vi "GUI_HTU_Control_Center.vi"() -> ()   [LabVIEW 2020]
uses:
  Shared/GUI_Template/GUI_master/tcp_new_data_event.ctl
  Shared/GUI_Template/GUI_master/tcp new data cluster.ctl
  GUI_TestStand/Fire button.ctl
panel:
  in  "Position.Ch1::36":dbl caption="TC Out Stage" min=0.0 max=12.0
  in  "Position.Ch2::36":dbl caption="TC In Stage" min=0.0 max=12.0
  in  "GUIdevice 36":string="U_EMQTripletBipolar"
  in  "DO.Ch21::22":enum16{"off", "on"}(ring) caption="UV spec\nmirror"
  in  "gaia shutter B":bool caption="Gaia internal\nshutter B"
  in  "gaia shutter A":bool caption="Gaia internal \nshutter A"
  in  "DO.Ch20::22":enum16{"off", "on"}(ring) caption="UV spec\nprotector"
  in  "Current_Limit.Ch4::35":dbl caption="BCave Trim\nCurrent" min=0.0 max=12.0
  in  "GUIdevice 35":string="U_EMQTripletBipolar"
  in  "Current::34":dbl caption="ACave \nCurrent" min=-40.0 max=40.0
  in  "Current_Limit.Ch1::33":dbl caption="BCave \nCurrent" min=0.0 max=120.0
  in  "GUIdevice 34":string="U_ACaveMagSpecPS"
  in  "GUIdevice 33":string="U_BCaveMagSpecPS"
  out "Rawfield::32":dbl caption="ACave Hall \nprobe" min=0.0 max=0.0
  in  "GUIdevice 32":string="U_ACaveHallProbe"
  out "Rawfield::31":dbl caption="BCave Hall \nprobe" min=0.0 max=0.0
  in  "GUIdevice 31":string="U_BCaveHallProbe"
  in  "Amplitude.Ch AB::30":dbl caption="Amplitude Jet trigger" min=0.5 max=5.0 format="%.1f"
  out "Amplitude.Ch AB::30":dbl caption="Amplitude\n Jet trigger" min=0.5 max=5.0 format="%.1f"
  in  "MRC trigger":bool caption="MRC \nTrigger"
  in  "GUIdevice 30":string="U_MRC_TimingBox"
  out "Internal Shutter B":string
  out "Internal Shutter A":string
  out "PockelCellB::29":dbl caption="pockelcellB" min=0.0 max=0.0 format="%.3f"
  out "pockelcella::29":dbl caption="pockelcellA" min=0.0 max=0.0 format="%.3f"
  in  "internalshutterb::29":dbl caption="Internal Shutter B" min=0.0 max=0.0 format="%.3f"
  in  "internalshuttera::29":dbl caption="Internal Shutter A" min=0.0 max=0.0 format="%.3f"
  in  "GUIdevice 29":string="U_GaiaSVEReader"
  in  "delay.Channel_C::18":dbl caption="Gaia lamp timing" min=-1.0 max=1.0
  in  "GUIdevice 18":string="U_1HzShiftedBox"
  in  "Position.Ch3::26":dbl caption="Ghost\nfilter" min=0.0 max=100.0
  in  "Position.Ch2::26":dbl caption="Ghost\nfocus" min=0.0 max=100.0
  in  "GUIdevice 15":string="U_MI_CoarseFilters"
  in  "GUIdevice 14":string="U_HASO_Filters"
  in  "GUIdevice 9":string="U_ProbeFilters"
  in  "DO.Ch11::22":enum16{"off", "on"}(ring) caption="TC phos"
  in  "GUIdevice 28":string="U_MI_FineFilters"
  in  "pos.Channel0::28":enum16{"1", "2", "3", "4", "5", "6"}(ring) caption="Fine Filters"
  in  "DO.Ch9::22":enum16{"off", "on"}(ring) caption="Aline2"
  in  "SoftwareVars.Ch1::22":enum16{"off", "on"}(ring) caption="Autopurge"
  in  "DO.Ch8::22":enum16{"off", "on"}(ring) caption="Aline 3"
  in  "DO.Ch7::22":enum16{"off", "on"}(ring) caption="DC Phos"
  in  "auto purge":bool=TRUE
  in  "purge":bool caption="Purge"
  in  "DO.Ch6::22":enum16{"off", "on"}(ring) caption="purge"
  in  "Offset::20":dbl caption="Probe cam\noffset" min=-40.0 max=40.0 format="%#_3g"
  out "AI_mean.Channel 1::27":dbl caption="Energy (nJ)" min=0.0 max=0.0 format="%.3f"
  out "AI_mean.Channel 0::27":dbl caption="Energy (nJ)" min=0.0 max=0.0 format="%.3f"
  in  "GUIdevice 27":string="U_VacuumGauge"
  out "ACavePressure":dbl format="%#_3g"
  out "BCavePressure":dbl format="%#_3g"
  in  "DO.Ch19::22":enum16{"off", "on"}(ring) caption="Visa9"
  in  "Position.Ch1::26":dbl caption="Phasics\nfocus" min=0.0 max=99.0
  in  "GUIdevice 26":string="U_Zaber"
  in  "DigitalOutput.Channel 7::25":enum16{"off", "on"}(ring) caption="Visa1"
  in  "DigitalOutput.Channel 6::25":enum16{"off", "on"}(ring) caption="Visa2"
  in  "DigitalOutput.Channel 5::25":enum16{"off", "on"}(ring) caption="Visa3"
  in  "DigitalOutput.Channel 4::25":enum16{"off", "on"}(ring) caption="Visa4"
  in  "DigitalOutput.Channel 3::25":enum16{"off", "on"}(ring) caption="Visa5"
  in  "DigitalOutput.Channel 2::25":enum16{"off", "on"}(ring) caption="Visa6"
  in  "DigitalOutput.Channel 1::25":enum16{"off", "on"}(ring) caption="Visa7"
  in  "DigitalOutput.Channel 0::25":enum16{"off", "on"}(ring) caption="Visa8"
  in  "GUIdevice 25":string="U_VisaPlungers"
  in  "DO.Ch18::22":enum16{"off", "on"}(ring) caption="Aline1"
  in  "GUIdevice 23":string="U_SSR_2"
  in  "DO.Ch5::22":enum16{"off", "on"}(ring) caption="Beam \nDump"
  in  "DO.Ch4::22":enum16{"off", "on"}(ring) caption="Phos1"
  in  "DO.Ch3::22":enum16{"off", "on"}(ring) caption="MI Wedge"
  in  "DO.Ch2::22":enum16{"off", "on"}(ring) caption="Slit"
  in  "DO.Ch1::22":enum16{"off", "on"}(ring) caption="OAPin2"
  in  "GUIdevice 22":string="U_PLC"
  in  "GUIdevice 21":string="U_BCavePicoServer"
  in  "Position::20":dbl caption="Probe cam\nStage" min=-25.0 max=25.0 format="%#_3g"
  in  "GUIdevice 20":string="U_ProbeCamStage"
  in  "Position.Axis 6::16":dbl caption="DM Surf. Y" min=1.9 max=3.0
  in  "Position.Axis 5::16":dbl caption="DM Surf. X" min=1.5 max=3.1
  in  "pos.Channel0::14":enum16{"1", "2", "3", "4", "5", "6"}(ring) caption="HASO"
  in  "pos.Channel0::19":enum16{"1", "2", "3", "4", "5", "6"}(ring) caption="Grating \nCam"
  in  "GUIdevice 19":string="U_FilterWheel_02"
  in  "Delay.Ch B::10":dbl caption="OPening time" min=0.0 max=0.1 format="%#_6p"
  in  "Amplitude.Ch AB::10":dbl caption="Amplitude Jet trigger" min=0.5 max=5.0 format="%.1f"
  in  "DO.Ch10::22":enum16{"off", "on"}(ring) caption="CTR"
  in  "GUIdevice 17":string="U_Hexapod"
  out "Position.Axis2::11":dbl caption="Angle 1" min=-180.0 max=180.0
  out "Position.Axis3::11":dbl caption="Angle 2" min=-180.0 max=180.0
  in  "Position.Axis 4::16":dbl caption="OAP1 In Y" min=2.0 max=5.0
  in  "Position.Axis 3::16":dbl caption="OAP1 In X" min=2.25 max=3.3
  in  "Position.Axis 2::16":dbl caption="BCave In Y" min=2.5 max=3.5
  in  "Position.Axis 1::16":dbl caption="BCave In X" min=2.0 max=4.0
  in  "GUIdevice 16":string="U_TRAServer03"
  in  "Position.Channel 9::1":T1(ring) caption="Amp 4 dump"
  in  "Position.Channel 10::1":T1(ring) caption="Gaia amp2 south energy"
  in  "Position.Axis 111::13":dbl caption="Blade Height" min=-999999.0 max=999999.0
  in  "GUIdevice 13":string="U_BCavePicoServer"
  in  "GUIdevice 12":string="U_TRAServer03"
  in  "Position.Channel 7::1":T1(ring) caption="Gaia Beamblock 2-North"
  in  "Position.Channel 8::1":T1(ring) caption="Gaia Beamblock 2-South"
  out "Delay.Ch B::10":dbl caption="Opening \ntime (s)" min=0.0 max=0.1 format="%#_6p"
  in  "Set opening time (s)":dbl
  in  "Jet enable":bool caption="Jet Enable"
  in  "Position.Axis 3::6":dbl caption="Probe \ndelay" min=0.0 max=25.0
  in  "Position.Axis 2::6":dbl caption="Jet Blade" min=-23.5 max=0.0
  in  "Position.Axis1::11":dbl caption="Separation" min=-60000.0 max=60000.0
  in  "GUIdevice 11":string="U_CompAerotech"
  in  "pos.Channel0::9":enum16{"1", "2", "3", "4", "5", "6"}(ring) caption="Probe"
  in  "pos.Channel0::5":enum16{"1", "2", "3", "4", "5", "6"}(ring) caption="Ghost\npulsed"
  in  "AnalogOutput.Channel 1::8":dbl caption="Pressure Control Voltage (V)" min=0.0 max=10.0
  in  "Position.Axis 3::7":dbl caption="Jet_Z" min=0.0 max=25.0
  in  "Position.Axis 2::7":dbl caption="Jet_Y" min=-25.0 max=0.0
  in  "Position.Axis 1::7":dbl caption="Jet_X" min=0.0 max=25.0
  in  "pos.Channel0::15":enum16{"1", "2", "3", "4", "5", "6"}(ring) caption="Coarse Filters"
  in  "Position.Channel 6::1":T1(ring) caption="Gaia Beamblock 3-North"
  in  "Position.Channel 5::1":T1(ring) caption="Gaia Beamblock 4-North"
  in  "Position.Channel 4::1":T1(ring) caption="Gaia Stop South"
  in  "Position.Channel 3::1":T1(ring) caption="Gaia Stop North"
  in  "Position.Channel 2::1":T1(ring) caption="Gaia Beamblock 3-South"
  in  "Position.Channel 1::1":T1(ring) caption="Gaia Beamblock 4-South"
  in  "Position.Axis 1::6":dbl caption="Position" min=-130.0 max=30.0
  in  "Position.Axis 6::4":dbl caption="Beamline In Y" min=1.5 max=2.9
  in  "Position.Axis 5::4":dbl caption="Beamline In X" min=2.5 max=4.0
  in  "Position.Axis 4::4":dbl caption="Beamline Out Y" min=2.6 max=3.2
  in  "Position.Axis 3::4":dbl caption="Beamline Out X" min=2.8 max=3.4
  in  "Position.Axis 2::4":dbl caption="OAP In 2 Y" min=2.5 max=3.3
  in  "Position.Axis 1::4":dbl caption="OAP In 2 X" min=3.1 max=3.6
  in  "Position.Axis 4::3":dbl caption="Comp In Y" min=5.5 max=5.9
  in  "Position.Axis 3::3":dbl caption="Comp In X" min=1.3 max=1.6
  in  "Position.Axis 2::3":dbl caption="Tube In Y" min=1.4 max=1.6
  in  "Position.Axis 1::3":dbl caption="Tube In X" min=1.2 max=1.4
  in  "GUIdevice 8":string="U_HP_Daq"
  in  "GUIdevice 6":string="U_ModeImagerESP"
  in  "GUIdevice 5":string="U_GhostFilters"
  in  "Fire Button":T2=TRUE
  out "error IO 2":errorcluster
  out "Amplitude.Ch AB::10":dbl caption="Amplitude\n Jet trigger" min=0.5 max=5.0 format="%.1f"
  out "fire::10":string
  out "tcp data event":T3
  in  "UDP error message":string
  in  "GUIdevice 7":string="U_ESP_JetXYZ"
  in  "GUIdevice 2":string="U_1Wire_Bcave"
  in  "GUIdevice 10":string="U_DG645_ShotControl"
  in  "GUIdevice 4":string="U_TRAServer02"
  in  "GUIdevice 1":string="U_1Wire_148"
  in  "GUIdevice 3":string="U_TRAServer01"
  in  "Step size":dbl min=-22.0 max=22.0 format="%.5f"
  in  "wangle::17":dbl caption="w" min=-7.5 max=7.5 step=0.01 format="%.5f"
  in  "vangle::17":dbl caption="v" min=-7.5 max=7.5 step=0.01 format="%.5f"
  in  "uangle::17":dbl caption="u" min=-7.5 max=7.5 step=0.01 format="%.5f"
  in  "ypos::17":dbl caption="y" min=-24.0 max=24.0 step=0.01 format="%.5f"
  in  "zpos::17":dbl caption="z" min=-10.0 max=10.0 step=0.01 format="%.5f"
  in  "xpos::17":dbl caption="x" min=-20.0 max=20.0 step=0.01 format="%.5f"
  in  "Jet trigger":bool caption="Jet Trigger"
  in  "Delay.Ch C::10":dbl caption="Jet timing (s)" min=-0.1 max=0.1 format="%#_6p"
  in  "stop":bool
  # "HTU CONTROL CENTER"
  # "Jet Stages"
  # "GAIA control"
  # "B-Cave Alignment"
  # "\"+x\" moves toward parking lot\n\"+y\" moves down\n\"+z\" moves upstream\n\"+\" moves jet blade out of jet\n\"+\" blade height moves away from jet"
  # "Mode Imager"
  # "Jet timing"
  # "Compressor"
  # "Hexapod"
  # "Misc area"
  # "148 TRA motors"
  # "\"+x\" is laser propagation direction\n\"+y\" is toward parking lot\n\"+z\" is up\nPMQ out at y=-22.0, in at ~17.5"
  # "\"in\" at position 0.0\n\"out\" at position 75.0"
  # "Vacuum"
  # "Valve Control"
  # "Extra Flippers"
  # "Mag Specs"
  # "Filters"
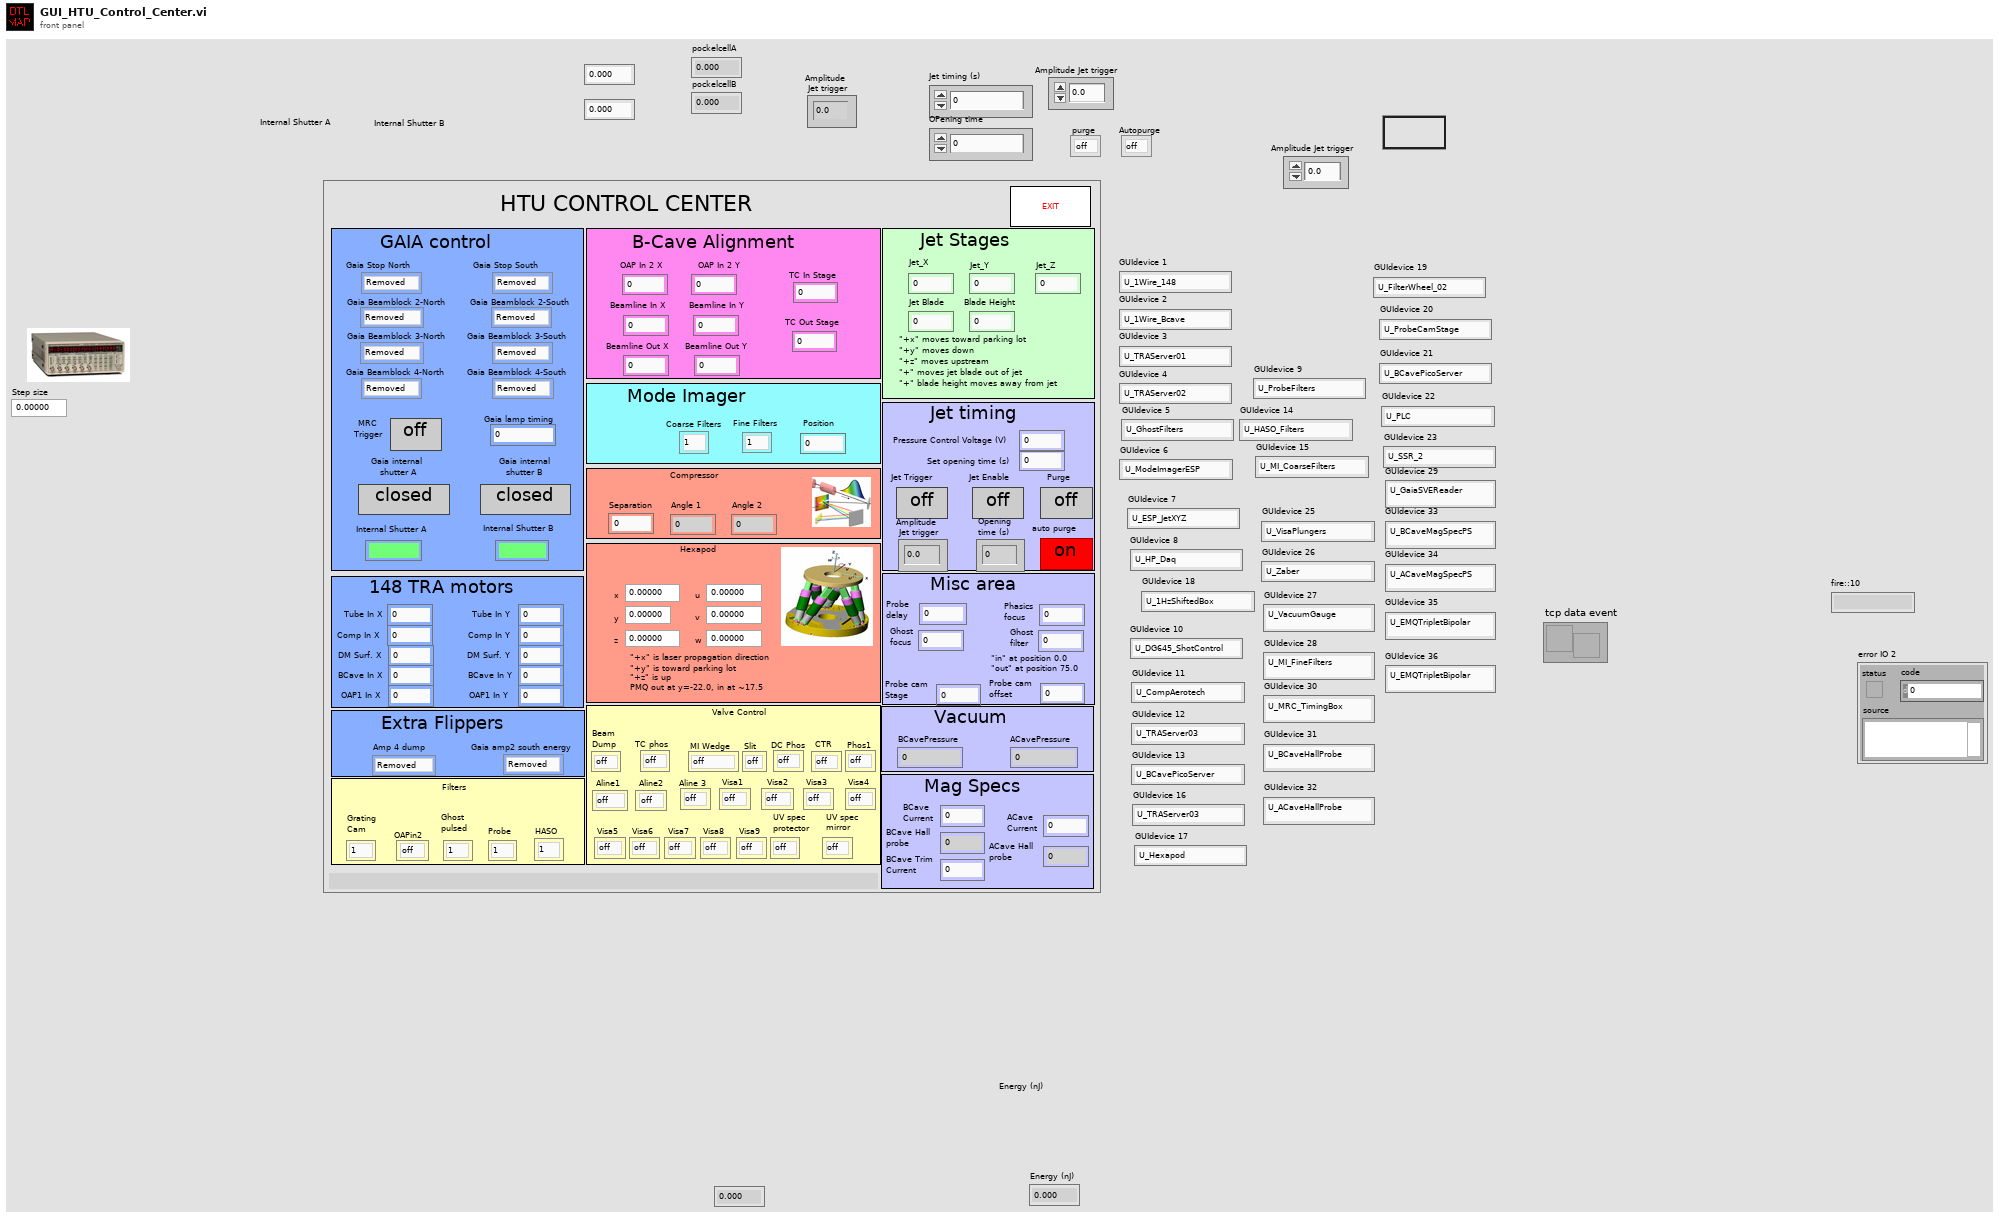
[diagram p1: front panel]
types:
  T1 = enum16{"Removed", "Inserted", "Unknown", "Moving"}
  T2 = typedef "Fire button.ctl" = bool
  T3 = typedef "tcp_new_data_event.ctl" = refnum<user-event>
  T4 = typedef "tcp new data cluster.ctl" = cluster{"EventEnum":enum16{"new data", "connection status update"}, "Device name":string}
  T5 = enum32{"invalid app kind", "Development System", "Run Time System", "Student Edition", "Embedded LabVIEW", "Evaluation", "Custom"}
  T6 = enum32{"Invalid", "Standard", "Closed", "Hidden", "Minimized", "Maximized"}
  T7 = cluster{"Core":cluster{"Current VI Reference":refnum<vi>, "Close Panel on Exit?":bool}, "BCavePressure":dbl, "ACavePressure":dbl, "Jet trigger":bool, "Jet probe stage tck":u32, "Tik2":u32, "Fire Continues Allowed":bool, "Jet enable":bool, "Wedge enable":bool, "Phosphor enable":bool, "jet status tck":i32, "purge":bool, "auto purge":bool, "MRC trigger":bool, "gaia shutter A":bool, "gaia shutter B":bool}
  T8 = cluster{"Current VI Reference":refnum<vi>, "Close Panel on Exit?":bool}
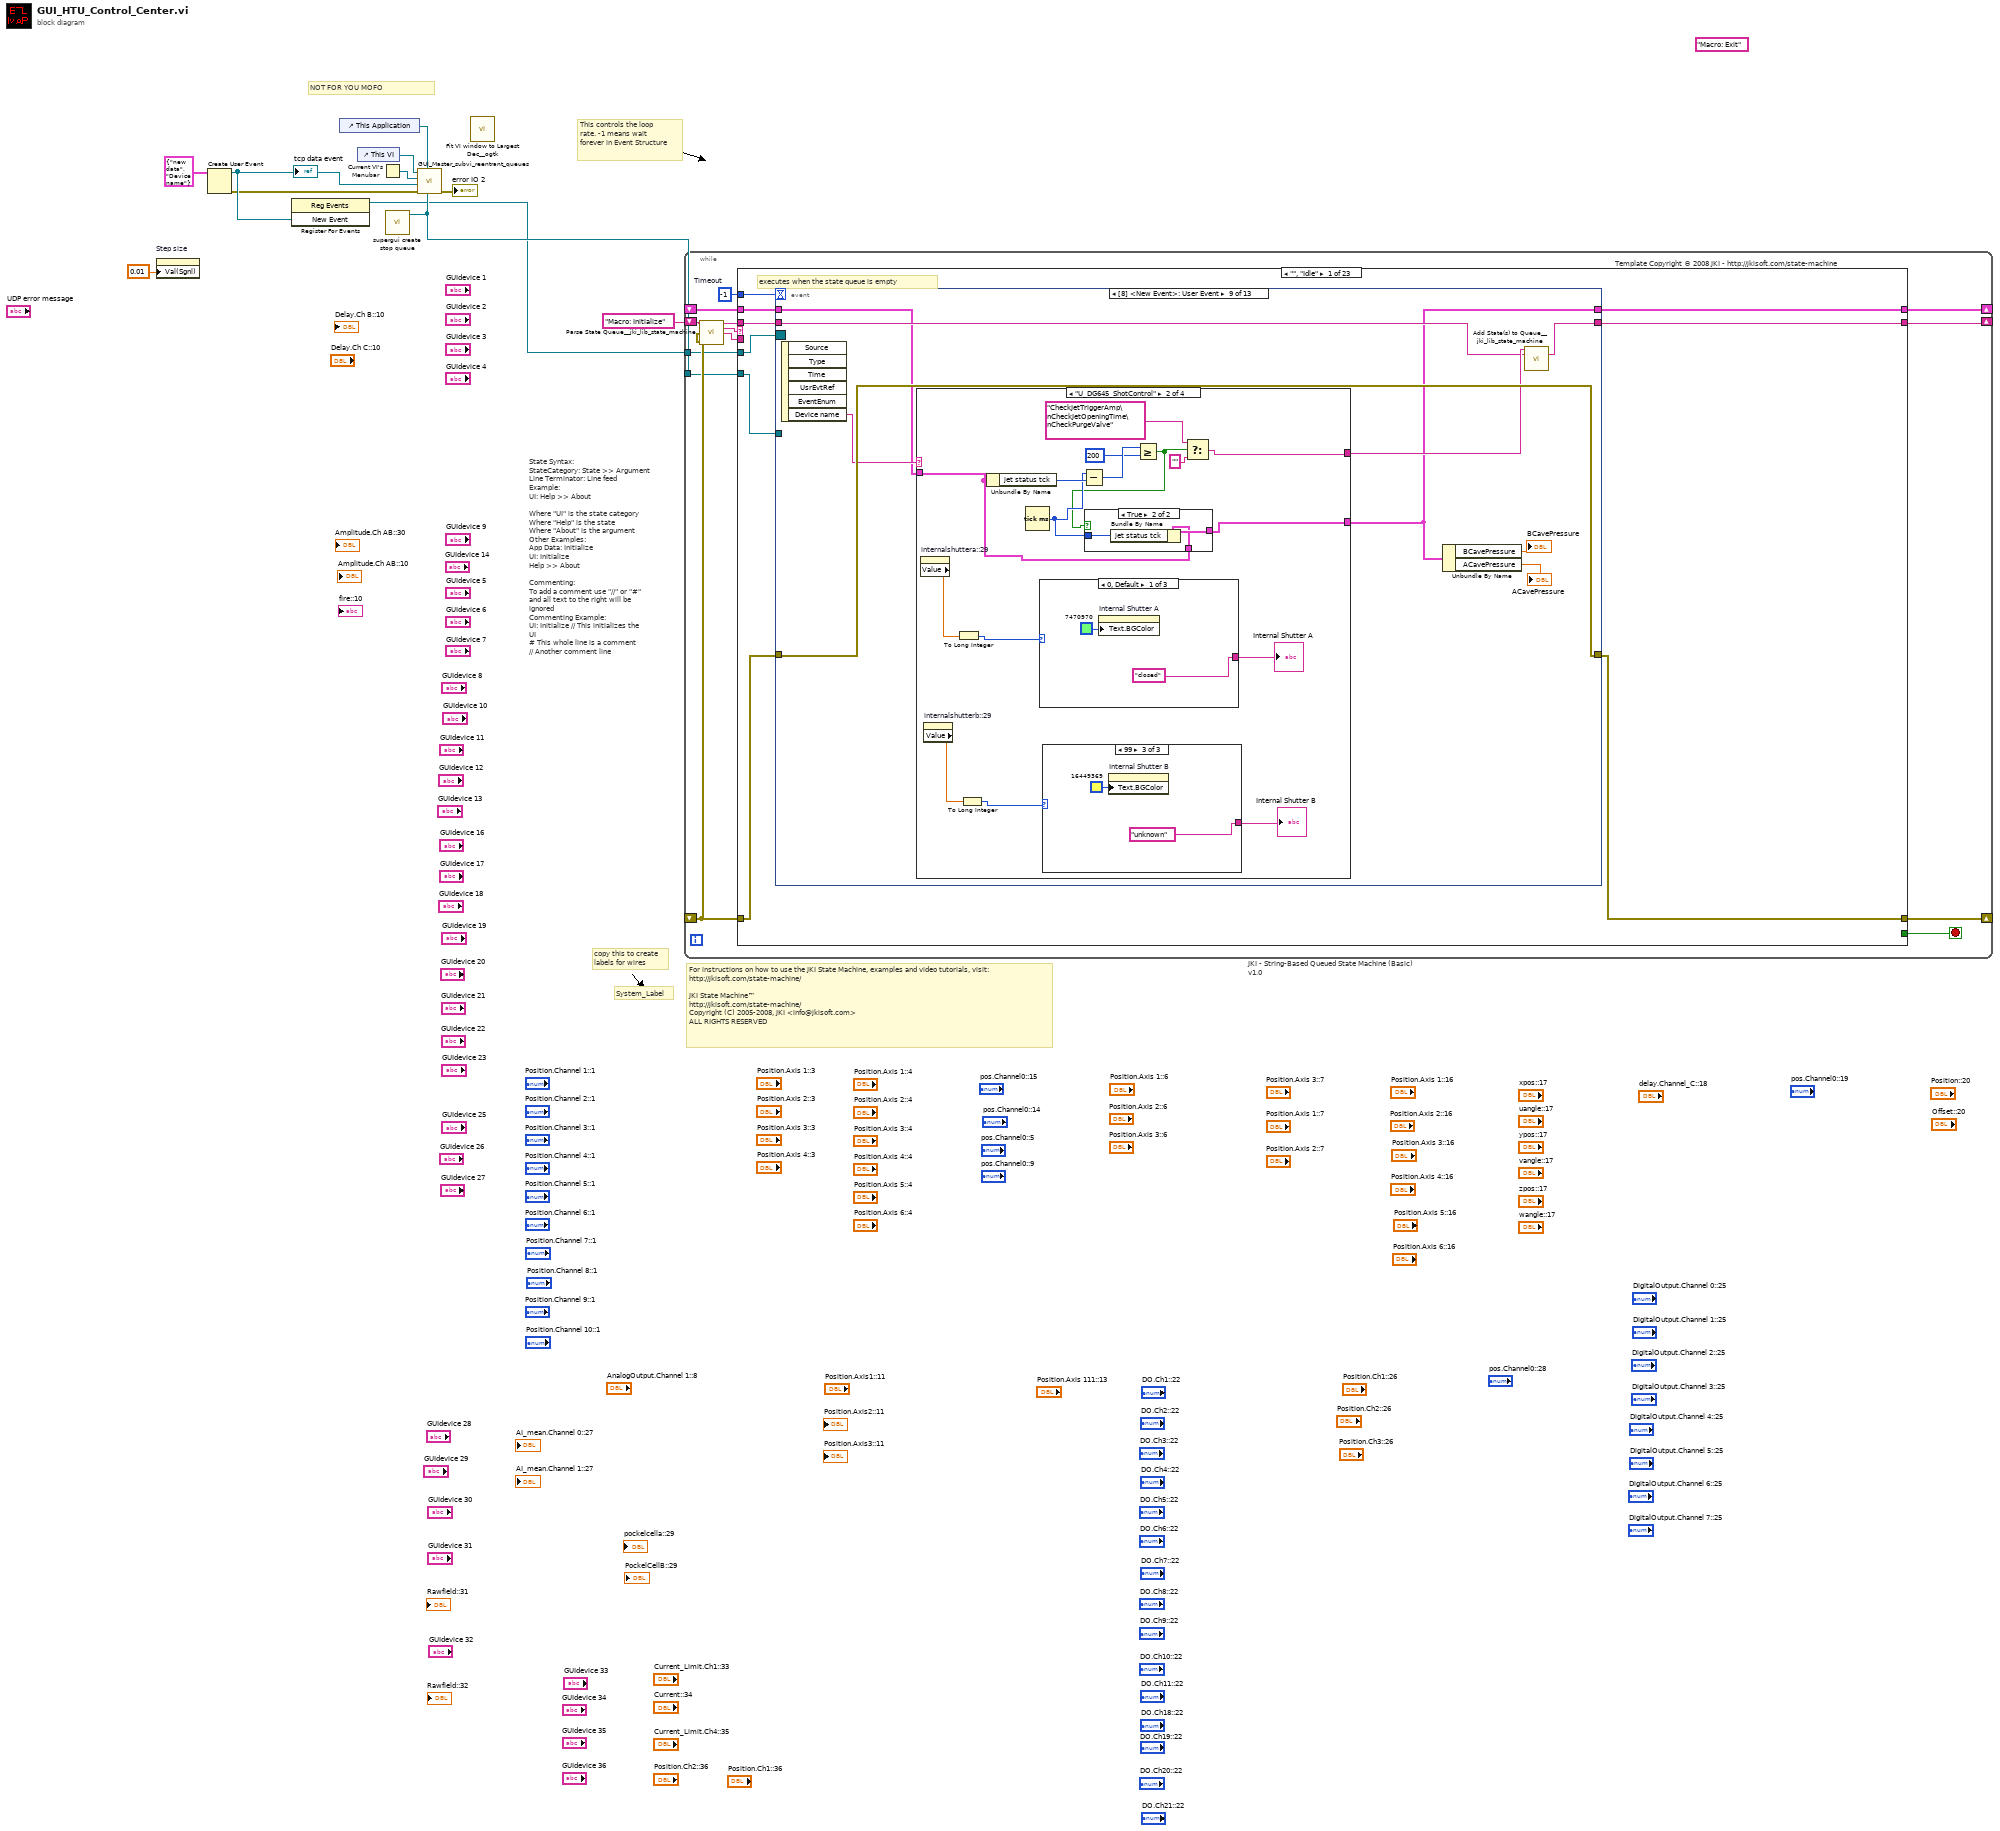
[diagram p0: block diagram]
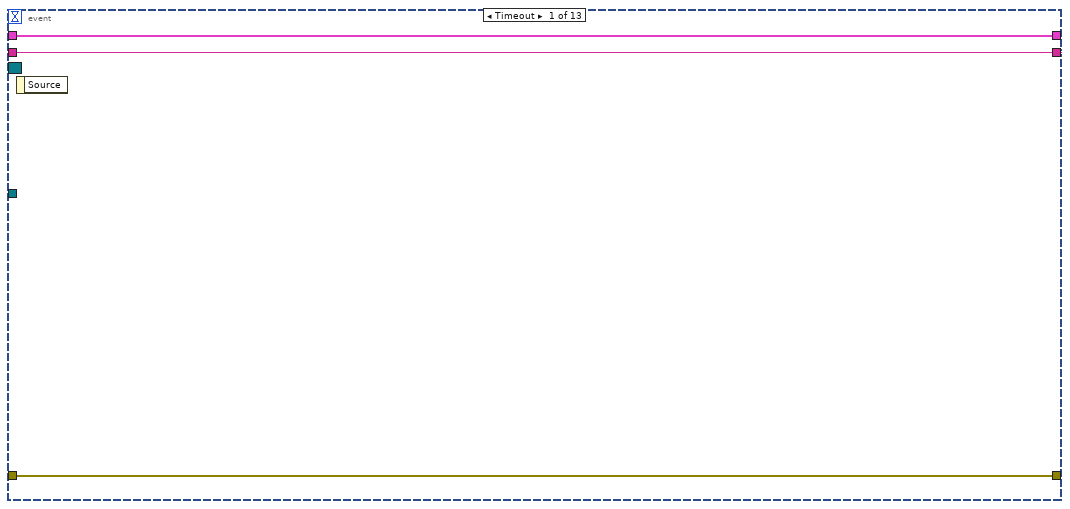
[diagram p2: hidden frame]
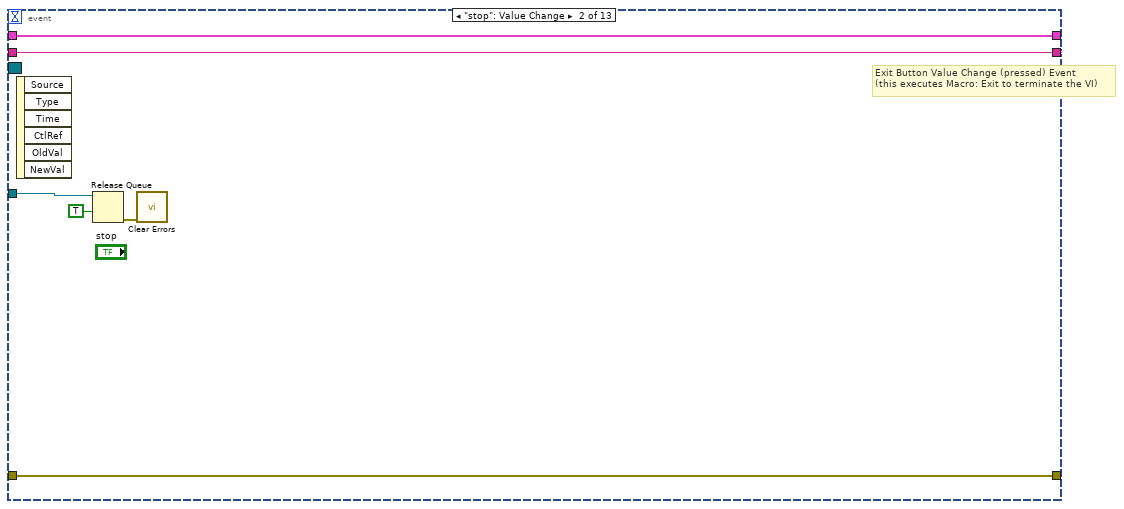
[diagram p3: hidden frame]
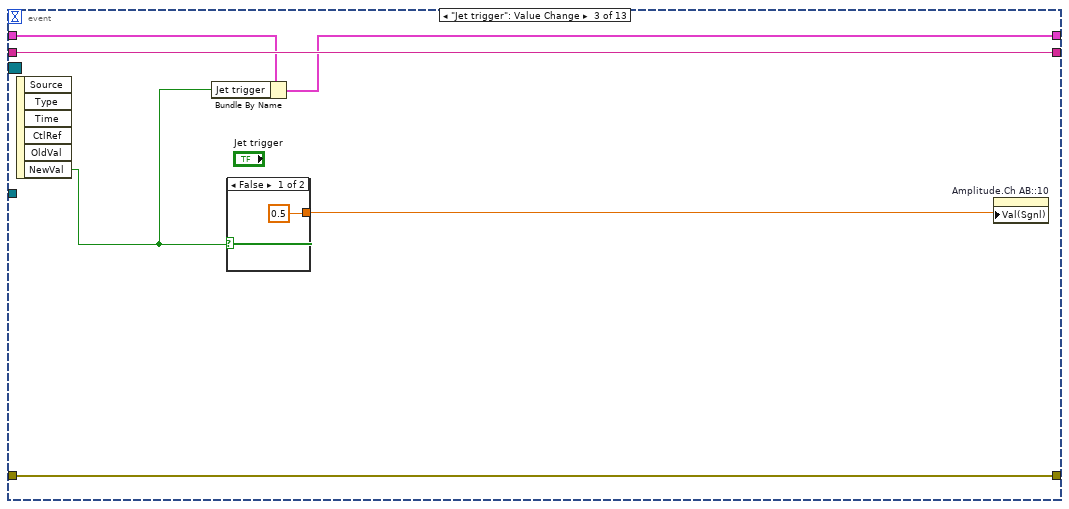
[diagram p4: hidden frame]
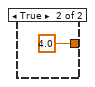
[diagram p5: hidden frame]
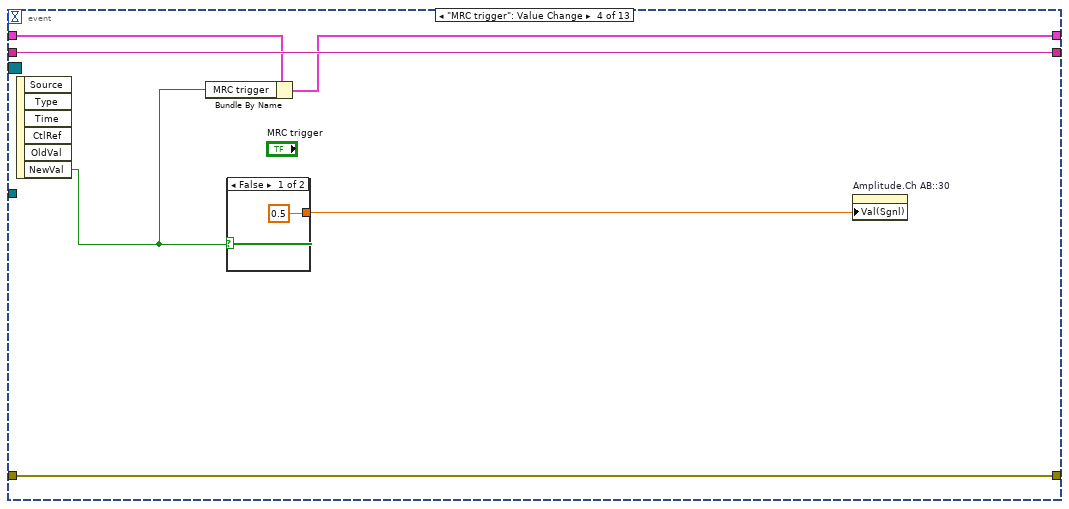
[diagram p6: hidden frame]
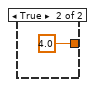
[diagram p7: hidden frame]
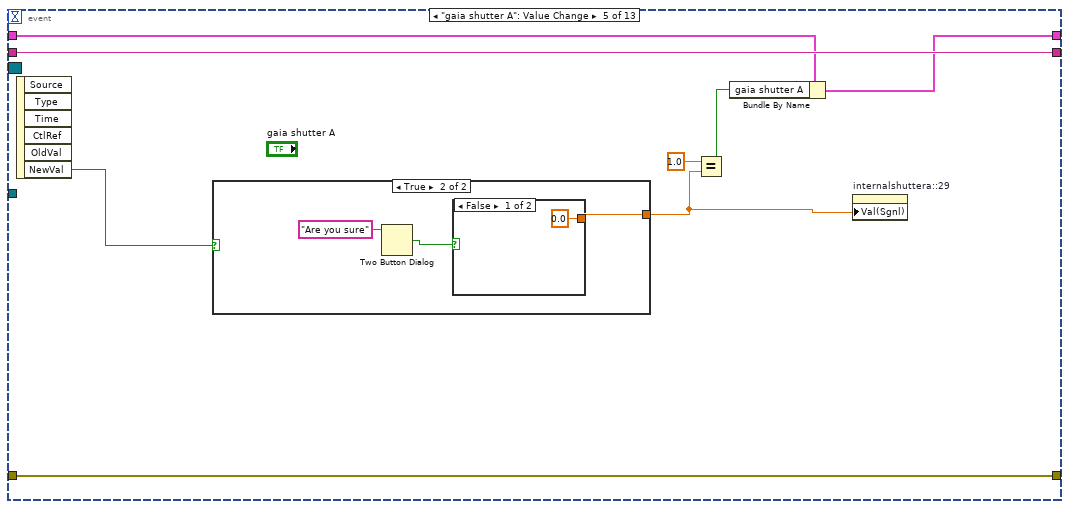
[diagram p8: hidden frame]
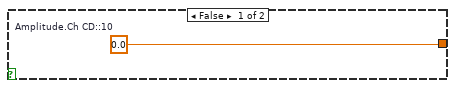
[diagram p9: hidden frame]
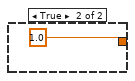
[diagram p10: hidden frame]
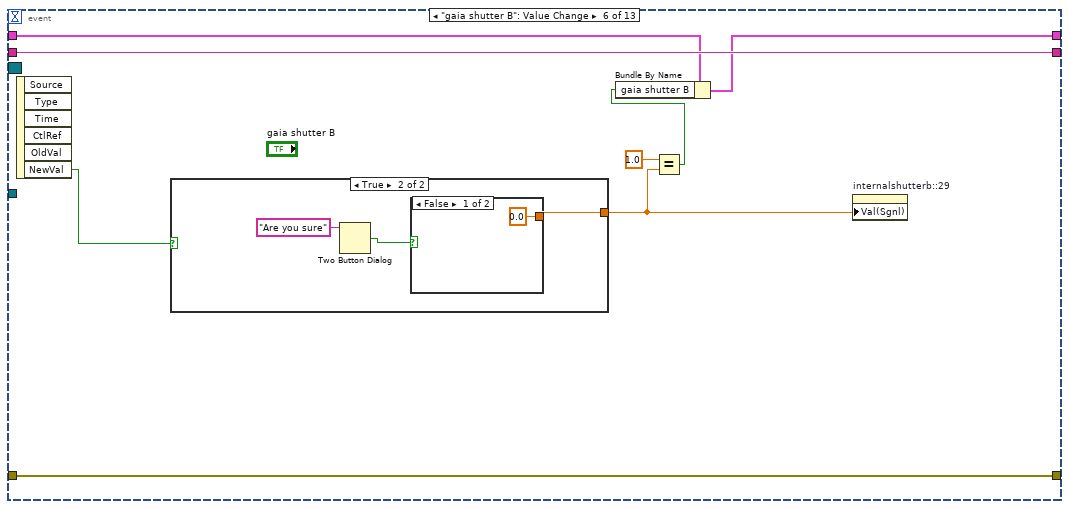
[diagram p11: hidden frame]
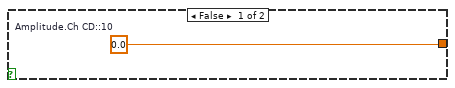
[diagram p12: hidden frame]
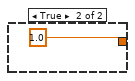
[diagram p13: hidden frame]
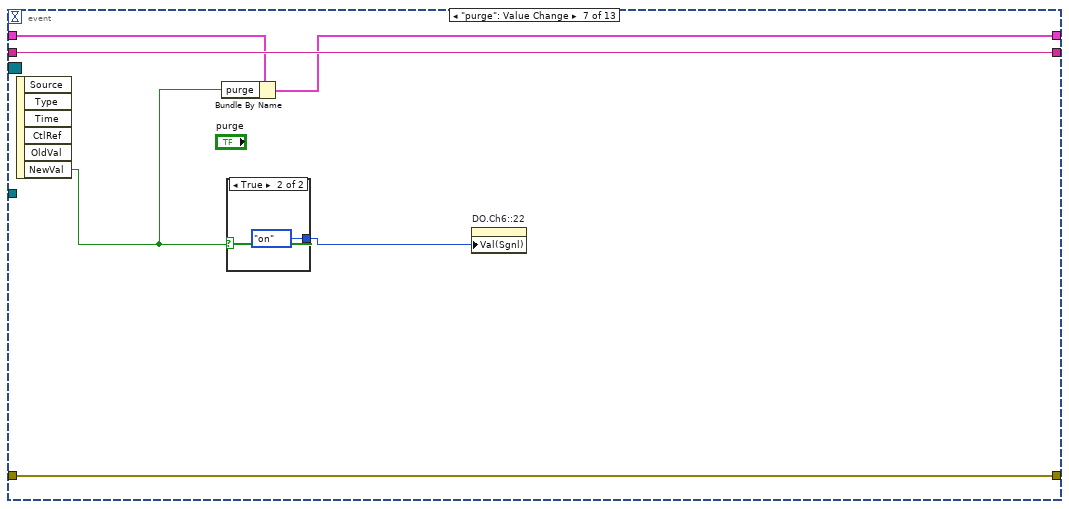
[diagram p14: hidden frame]
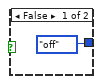
[diagram p15: hidden frame]
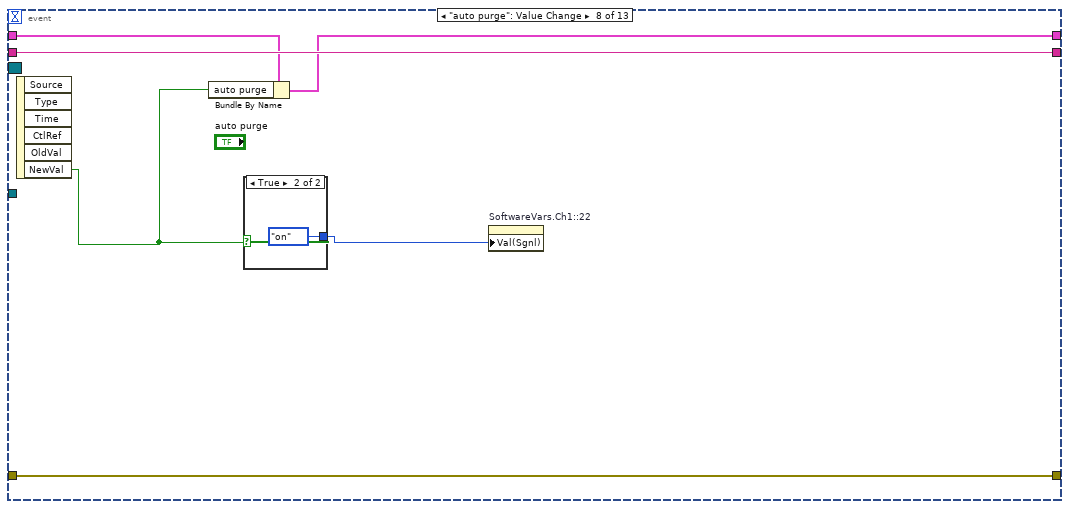
[diagram p16: hidden frame]
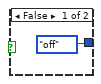
[diagram p17: hidden frame]
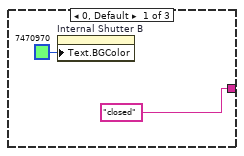
[diagram p19: hidden frame]
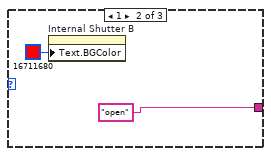
[diagram p20: hidden frame]
diagram:
  (unwired) "Macro: Exit"
  # "For instructions on how to use the JKI State Machine, examples and video tutorials, visit:\nhttp://jkisoft.com/state-machine/\n\nJKI State Machine™\nhttp://jkisoft.com/state-machine/\nCopyright (C) 2005-2008, JKI <info@jkisoft.com>\nALL RIGHTS RESERVED"
  # "State Syntax:\nStateCategory: State >> Argument\nLine Terminator: Line feed\nExample:\nUI: Help >> About\n\nWhere \"UI\" is the state category\nWhere \"Help\" is the state\nWhere \"About\" is the argument\nOther Examples:\nApp Data: Initialize\nUI: Initialize\nHelp >> About\n\nCommenting:\nTo add a comment use \"//\" or \"#\" and all text to the right will be ignored\nCommenting Example:\nUI: Initialize // This initializes the UI\n# This whole line is a comment\n// Another comment line"
  # "copy this to create labels for wires"
  # "This controls the loop rate. -1 means wait forever in Event Structure"
  # "System_Label"
  # "NOT FOR YOU MOFO"
  n1 = property on="Step size" class="DigNum (strict)"("Val(Sgnl)"=0.01 ("Value (Signaling)")) -> ()  [unwired: 2 in, 2 out]
  n2 = Create User Event(user event datatype=T4 {"EventEnum"=enum."new data", "Device name"="Device name"} ("New Event")) -> (user event=w10:refnum<user-event>, error out=w9:errorcluster)  [unwired: 1 in]
  "tcp data event" <- w10
  n3 = register-events(w10) -> (reference out=w1:refnum<event-registration>)  [unwired: 2 in, 1 out]
  n4 = control-ref of="This Application"() -> (w11:refnum<vi>)
  n5 = control-ref of="This VI"() -> (w4:refnum<vi>)
  n6 = Current VI's Menubar() -> (w7:refnum<k9>)
  n7 = call "supergui create stop queue.vi"() -> ("STOP Queue out"=w2:refnum<queue>)  [unwired: 11 in]
  n8 = call "GUI_Master_subvi_reentrant_queues.vi"("STOP Queue in"=w2, "This Application"=w11, "error in (no error)"=w9, "tcp data event"=w10, "Caller menu reference"=w7, "Caller VI ref"=w4) -> ("error out"=→"error IO 2":errorcluster)  [unwired: 5 in]
  n9 = call <userlib>:"Fit VI window to Largest Dec__ogtk.vi"() -> ()  [unwired: 6 in, 2 out]
  n10 = while "JKI - String-Based Queued State Machine (Basic) v1.0" {
    shift-right: [w17] -> _
    shift-left: _ -> [w16]
    shift-right: [w20] -> _
    shift-left: _ -> [w14]
    shift-right: [w19] -> _
    shift-left: "Macro: Initialize" -> [w21]
    tunnel: w1 -> [w13]
    tunnel: w2 -> [w12]
    stop <- w18 stop-if-true
    w15 = -1  # Timeout
    # "Template Copyright © 2008 JKI - http://jkisoft.com/state-machine"
    n11 = call <vilib>:"Parse State Queue__jki_lib_state_machine.vi"("State Queue"=w21, "Error In (no error)"=w14) -> ("Remaining States"=w23:string, "Current State"=w24:string, "Arguments"=w22:string)  [unwired: 11 in]
    n12 = case shown="\"\", \"Idle\"" w24 {
      selector: w24 -> [_ _ w203 _ _ _ _ _ _ _ _ _ _ _ _ _ _ _ _ _ _ _ _]
      tunnel: w23 -> [w33 w202 w207 w225 w231 w236 w240 w260 w266 w270 w274 w280 w291 w317 w322 w332 w336 w342 w367 w385 w402 w419 w471]
      tunnel: w22 -> [_ _ _ _ _ _ _ _ _ _ _ w275 w285 _ _ _ _ _ _ _ _ _ _]
      tunnel: w16 -> [w31 w199 w205 w216 w228 w234 w237 _ w261 w267 w272 w278 w287 w314 w319 w329 w333 w340 w364 w382 w399 w415 w460]
      tunnel: [w30 w200 w209 w222 errorcluster {"status"=FALSE, "code"=0, "source"=""} ("error out") w233 w238 w257 w262 w268 w271 w276 w288 w315 w320 w330 w334 w337 w365 w383 w398 w412 w461] -> w20
      tunnel: w14 -> [w25 w200 w208 w222 w227 w233 w238 w257 w263 w268 w271 w277 w289 w315 w320 w330 w334 w338 w365 w383 w396 w413 w461]
      tunnel: [w32 w201 w206 w224 w230 w235 w239 w259 w265 w269 w273 w279 w290 w316 w321 w331 w335 w341 w366 w384 w401 w418 w470] -> w19
      tunnel: [_ _ _ _ _ TRUE _ _ _ _ _ _ _ _ _ _ _ _ _ _ _ _ _] -> w18
      tunnel: [w26 w199 w205 w223 w228 w234 w237 w258 w261 w267 w272 w278 w287 w314 w319 w329 w333 w340 w363 w381 w399 w414 w459] -> w17
      tunnel: w15 -> [w29 _ _ _ _ _ _ _ _ _ _ _ _ _ _ _ _ _ _ _ _ _ _]
      tunnel: w13 -> [w28 _ _ _ _ _ _ _ _ _ _ _ _ _ _ _ _ _ _ _ _ _ _]
      tunnel: w12 -> [w27 _ _ _ _ _ _ _ _ _ _ _ _ _ _ _ _ _ _ _ _ _ _]
      frame "", "Idle" {
        # "executes when the state queue is empty"
        n13 = event shown="[8] <New Event>: User Event" {
          selector: w28 -> [_ _ _ _ _ _ _ _ _ _ _ _ _]
          dyn-events: _ -> [_ _ _ _ _ _ _ _ _ _ _ _ _]
          timeout: w29 -> [_ _ _ _ _ _ _ _ _ _ _ _ _]
          tunnel: w33 -> [w37 w45 w51 w59 w69 w83 w95 w103 w111 w181 w185 w190 w198]
          tunnel: [w36 w44 w51 w59 w69 w83 w95 w103 w110 w181 w186 w190 w197] -> w32
          tunnel: w31 -> [w34 w42 w50 w58 w68 w82 w94 w102 w109 w180 w188 w191 w195]
          tunnel: [w35 w43 w46 w54 w66 w79 w91 w100 w114 w176 w187 w189 w196] -> w30
          tunnel: w25 -> [w35 w43 w46 w54 w66 w79 w91 w100 w114 w176 w187 w189 w196]
          tunnel: [w34 w42 w49 w57 w67 w81 w93 w101 w108 w179 w188 w191 w195] -> w26
          tunnel: w27 -> [_ w39 _ _ _ _ _ _ _ _ _ _ _]
          event Timeout {
            n14 = event-data() -> ()  [unwired: 1 in, 1 out]
            n15 = call <vilib>:"Add State(s) to Queue__jki_lib_state_machine.vi"("State(s) in (\"\")"=w37) -> ("States Out"=w36:string)  [unwired: 14 in]
          }
          event "stop": Value Change {
            # "Exit Button Value Change (pressed) Event\n(this executes Macro: Exit to terminate the VI)"
            n16 = event-data() -> ()  [unwired: 1 in, 6 out]
            n17 = Release Queue(queue=w39, force destroy? (F)=TRUE) -> (error out=w40:errorcluster)  [unwired: 1 in, 2 out]
            n18 = call <vilib>:"Clear Errors.vi"("error in (no error)"=w40) -> ()  [unwired: 5 in, 2 out]
            n19 = call <vilib>:"Add State(s) to Queue__jki_lib_state_machine.vi"("State(s) in Front (\"\")"="Macro: Exit", "State(s) in (\"\")"=w45) -> ("States Out"=w44:string)  [unwired: 13 in]
          }
          event "Jet trigger": Value Change {
            n20 = event-data() -> ("NewVal"=w48:bool)  [unwired: 1 in, 5 out]
            n21 = Bundle By Name(cluster=w50, "Jet trigger"=w48) -> (w49:T7)
            n22 = case shown="False" w48 {
              tunnel: [0.5 ("Amplitude.Ch CD::10") 4.0 ("Amplitude.Ch CD::10")] -> w47
              frame False {
              }
              frame True {
              }
            }
            n23 = property on="Amplitude.Ch AB::10" class="DigNum (strict)"("Val(Sgnl)"=w47) -> ()  [unwired: 2 in, 2 out]
          }
          event "MRC trigger": Value Change {
            n24 = event-data() -> ("NewVal"=w56:bool)  [unwired: 1 in, 5 out]
            n25 = Bundle By Name(cluster=w58, "MRC trigger"=w56) -> (w57:T7)
            n26 = case shown="False" w56 {
              tunnel: [0.5 ("Amplitude.Ch CD::10") 4.0 ("Amplitude.Ch CD::10")] -> w55
              frame False {
              }
              frame True {
              }
            }
            n27 = property on="Amplitude.Ch AB::30" class="DigNum (strict)"("Val(Sgnl)"=w55) -> ()  [unwired: 2 in, 2 out]
          }
          event "gaia shutter A": Value Change {
            n28 = event-data() -> ("NewVal"=w63:bool)  [unwired: 1 in, 5 out]
            n29 = case shown="True" w63 {
              tunnel: [w70 w73] -> w64
              frame False {
                w70 = 0.0  # Amplitude.Ch CD::10
              }
              frame True {
                n30 = Two Button Dialog(message="Are you sure") -> (T button?=w71:bool)  [unwired: 2 in]
                n31 = case shown="False" w71 {
                  tunnel: [0.0 ("Amplitude.Ch CD::10") 1.0 ("Amplitude.Ch CD::10")] -> w73
                  frame False {
                  }
                  frame True {
                  }
                }
              }
            }
            n32 = Equal?(x=1.0, y=w64) -> (x = y?=w62:bool)
            n33 = Bundle By Name(cluster=w68, "gaia shutter A"=w62) -> (w67:T7)
            n34 = property on="internalshuttera::29" class="DigNum (strict)"("Val(Sgnl)"=w64) -> ()  [unwired: 2 in, 2 out]
          }
          event "gaia shutter B": Value Change {
            n35 = event-data() -> ("NewVal"=w80:bool)  [unwired: 1 in, 5 out]
            n36 = case shown="True" w80 {
              tunnel: [w84 w87] -> w78
              frame False {
                w84 = 0.0  # Amplitude.Ch CD::10
              }
              frame True {
                n37 = Two Button Dialog(message="Are you sure") -> (T button?=w85:bool)  [unwired: 2 in]
                n38 = case shown="False" w85 {
                  tunnel: [0.0 ("Amplitude.Ch CD::10") 1.0 ("Amplitude.Ch CD::10")] -> w87
                  frame False {
                  }
                  frame True {
                  }
                }
              }
            }
            n39 = Equal?(x=1.0, y=w78) -> (x = y?=w76:bool)
            n40 = Bundle By Name(cluster=w82, "gaia shutter B"=w76) -> (w81:T7)
            n41 = property on="internalshutterb::29" class="DigNum (strict)"("Val(Sgnl)"=w78) -> ()  [unwired: 2 in, 2 out]
          }
          event "purge": Value Change {
            n42 = event-data() -> ("NewVal"=w92:bool)  [unwired: 1 in, 5 out]
            n43 = Bundle By Name(cluster=w94, "purge"=w92) -> (w93:T7)
            n44 = case shown="True" w92 {
              tunnel: [enum16{"off", "on"}."off" ("Value (Signaling)") enum16{"off", "on"}."on" ("Value (Signaling)")] -> w90
              frame False {
              }
              frame True {
              }
            }
            n45 = property on="DO.Ch6::22" class="Enum (strict)"("Val(Sgnl)"=w90) -> ()  [unwired: 2 in, 2 out]
          }
          event "auto purge": Value Change {
            n46 = event-data() -> ("NewVal"=w98:bool)  [unwired: 1 in, 5 out]
            n47 = Bundle By Name(cluster=w102, "auto purge"=w98) -> (w101:T7)
            n48 = case shown="True" w98 {
              tunnel: [enum16{"off", "on"}."off" ("Value (Signaling)") enum16{"off", "on"}."on" ("Value (Signaling)")] -> w99
              frame False {
              }
              frame True {
              }
            }
            n49 = property on="SoftwareVars.Ch1::22" class="Enum (strict)"("Val(Sgnl)"=w99) -> ()  [unwired: 2 in, 2 out]
          }
          event User Event {
            n50 = event-data() -> ("Device name"=w113:string)  [unwired: 1 in, 5 out]
            n51 = case shown="\"U_DG645_ShotControl\"" w113 {
              tunnel: [_ w125 w149 w162] -> w112
              tunnel: w109 -> [w115 w123 w153 w164]
              tunnel: [w115 w122 w152 w163] -> w108
              frame "False", Default {
              }
              frame "U_DG645_ShotControl" {
                n52 = property on="internalshuttera::29" class="DigNum (strict)"() -> ("Value"=w116:dbl)  [unwired: 2 in, 2 out]
                n53 = property on="internalshutterb::29" class="DigNum (strict)"() -> ("Value"=w119:dbl)  [unwired: 2 in, 2 out]
                n54 = To Long Integer(number=w116) -> (32bit integer=w117:i32)
                n55 = To Long Integer(number=w119) -> (32bit integer=w120:i32)
                n56 = Unbundle By Name(w123) -> ("jet status tck"=w131:i32)
                n57 = Tick Count (ms)() -> (millisecond timer value=w127:u32)
                n58 = case shown="0, Default" w117 {
                  tunnel: ["closed" ("String") "open" ("String") "unknown" ("String")] -> w118
                  frame 0, Default {
                    n59 = property on="Internal Shutter A" class="Str"("Text.BGColor"=u32 7470970 ("Text.Text Colors:BG Color")) -> ()  [unwired: 2 in, 2 out]
                  }
                  frame 1 {
                    n60 = property on="Internal Shutter A" class="Str"("Text.BGColor"=u32 16711680 ("Text.Text Colors:BG Color")) -> ()  [unwired: 2 in, 2 out]
                  }
                  frame 99 {
                    n61 = property on="Internal Shutter A" class="Str"("Text.BGColor"=u32 16449369 ("Text.Text Colors:BG Color")) -> ()  [unwired: 2 in, 2 out]
                  }
                }
                "Internal Shutter A" <- w118
                n62 = case shown="99" w120 {
                  tunnel: ["closed" ("String") "open" ("String") "unknown" ("String")] -> w121
                  frame 0, Default {
                    n63 = property on="Internal Shutter B" class="Str"("Text.BGColor"=u32 7470970 ("Text.Text Colors:BG Color")) -> ()  [unwired: 2 in, 2 out]
                  }
                  frame 1 {
                    n64 = property on="Internal Shutter B" class="Str"("Text.BGColor"=u32 16711680 ("Text.Text Colors:BG Color")) -> ()  [unwired: 2 in, 2 out]
                  }
                  frame 99 {
                    n65 = property on="Internal Shutter B" class="Str"("Text.BGColor"=u32 16449369 ("Text.Text Colors:BG Color")) -> ()  [unwired: 2 in, 2 out]
                  }
                }
                "Internal Shutter B" <- w121
                n66 = Subtract(x=w127, y=w131) -> (x-y=w130:u32)
                n67 = Greater Or Equal?(x=w130, y=u32 200 ("x")) -> (x >= y?=w126:bool)
                n68 = case shown="True" w126 {
                  tunnel: [w144 w147] -> w122
                  tunnel: w123 -> [w144 w146]
                  tunnel: w127 -> [_ w145]
                  frame False {
                  }
                  frame True {
                    n69 = Bundle By Name(cluster=w146, "jet status tck"=w145) -> (w147:T7)
                  }
                }
                n70 = Select(t="CheckJetTriggerAmp\nCheckJetOpeningTime\nCheckPurgeValve", s=w126, f="") -> (s? t:f=w125:string)
              }
              frame "U_ESP_JetXYZ" {
                n71 = Unbundle By Name(w153) -> ("Jet probe stage tck"=w157:u32)
                n72 = Tick Count (ms)() -> (millisecond timer value=w154:u32)
                n73 = Subtract(x=w154, y=w157) -> (x-y=w156:u32)
                n74 = Greater Or Equal?(x=w156, y=u32 200 ("x")) -> (x >= y?=w148:bool)
                n75 = case shown="True" w148 {
                  tunnel: [w158 w161] -> w152
                  tunnel: w153 -> [w158 w160]
                  tunnel: w154 -> [_ w159]
                  frame False {
                  }
                  frame True {
                    n76 = Bundle By Name(cluster=w160, "Jet probe stage tck"=w159) -> (w161:T7)
                  }
                }
                n77 = Select(t="CheckProbeCamStage", s=w148, f="") -> (s? t:f=w149:string)
              }
              frame "U_VacuumGauge" {
                n78 = Unbundle By Name(w164) -> ("Jet probe stage tck"=w168:u32)
                n79 = Tick Count (ms)() -> (millisecond timer value=w170:u32)
                n80 = Subtract(x=w170, y=w168) -> (x-y=w169:u32)
                n81 = Greater Or Equal?(x=w169, y=u32 200 ("x")) -> (x >= y?=w171:bool)
                n82 = case shown="True" w171 {
                  tunnel: [w172 w175] -> w163
                  tunnel: w164 -> [w172 w174]
                  tunnel: w170 -> [_ w173]
                  frame False {
                  }
                  frame True {
                    n83 = Bundle By Name(cluster=w174, "Jet probe stage tck"=w173) -> (w175:T7)
                  }
                }
                n84 = Select(t="UpdatePressure", s=w171, f="") -> (s? t:f=w162:string)
              }
            }
            n85 = Unbundle By Name(w108) -> ("BCavePressure"=→"BCavePressure":dbl, "ACavePressure"=→"ACavePressure":dbl)
            n86 = call <vilib>:"Add State(s) to Queue__jki_lib_state_machine.vi"("State(s) in Front (\"\")"=w112, "State(s) in (\"\")"=w111) -> ("States Out"=w110:string)  [unwired: 13 in]
          }
          event "Jet enable": Value Change {
            n87 = event-data() -> ("NewVal"=w178:bool)  [unwired: 1 in, 5 out]
            n88 = case shown="True" w178 {
              tunnel: [0.0 ("opening Time") "Set opening time (s)"] -> w177
              frame False {
              }
              frame True {
              }
            }
            n89 = Bundle By Name(cluster=w180, "Jet enable"=w178) -> (w179:T7)
            n90 = property on="Delay.Ch B::10" class="DigNum (strict)"("Val(Sgnl)"=w177) -> ()  [unwired: 2 in, 2 out]
          }
          event Value Change {
            n91 = event-data() -> ()  [unwired: 1 in, 6 out]
            n92 = call <vilib>:"Add State(s) to Queue__jki_lib_state_machine.vi"("State(s) in Front (\"\")"="Action: Fire" ("State(s) in Front (\"\")"), "State(s) in (\"\")"=w185) -> ("States Out"=w186:string)  [unwired: 13 in]
          }
          event "Step size": Value Change {
            n93 = event-data() -> ("NewVal"=w192:dbl)  [unwired: 1 in, 5 out]
            n94 = property on="uangle::17" class="DigNum (strict)"("Increment"=w192) -> ()  [unwired: 2 in, 2 out]
            n95 = property on="vangle::17" class="DigNum (strict)"("Increment"=w192) -> ()  [unwired: 2 in, 2 out]
            n96 = property on="xpos::17" class="DigNum (strict)"("Increment"=w192) -> ()  [unwired: 2 in, 2 out]
            n97 = property on="zpos::17" class="DigNum (strict)"("Increment"=w192) -> ()  [unwired: 2 in, 2 out]
            n98 = property on="wangle::17" class="DigNum (strict)"("Increment"=w192) -> ()  [unwired: 2 in, 2 out]
            n99 = property on="ypos::17" class="DigNum (strict)"("Increment"=w192) -> ()  [unwired: 2 in, 2 out]
          }
          event Panel Close? {
            # "Discard the event because we'll close the front panel ourselves in Macro: Exit"
            # "Close Panel button (pressed) Event\n(this executes Macro: Exit to terminate the VI)"
            n100 = event-data() -> ()  [unwired: 1 in, 1 out]
            n101 = event-data("Discard?"=TRUE) -> ()  [unwired: 1 in, 1 out]
            n102 = call <vilib>:"Add State(s) to Queue__jki_lib_state_machine.vi"("State(s) in Front (\"\")"="Macro: Exit", "State(s) in (\"\")"=w198) -> ("States Out"=w197:string)  [unwired: 13 in]
          }
        }
      }
      frame "---------- Core ----------" {
        # "Do not put any code in this frame.\n(it is a separator no-op)"
        n103 = call <vilib>:"Add State(s) to Queue__jki_lib_state_machine.vi"("State(s) in (\"\")"=w202) -> ("States Out"=w201:string)  [unwired: 14 in]
      }
      frame Default {
        w212 = 42 items=["No error", "Argument error", "Memory is full", "Out of zone", "End of file", "File already open", "Generic file I/O error", "File not found", "File permission error", "Disk is full", "Duplicate path", "Too many files open", "System feature not enabled", "Resource file not found", "Cannot add resource", "Resource not found", "Image not found", "Image memory error", "Pen does not exist", "Config type invalid", "Config token not found", "Config parse error", "Config memory error", "Bad external code format", "Bad external code offset", "External code not present", "Null window", "Destroy window error", "Null menu", "Print aborted", "Bad print record", "Print driver error", "Windows error during printing", "Memory error during printing", "Print dialog error", "Generic print error", "Invalid device refnum", "Device not found", "Device parameter error", "Device unit error", "Cannot open device", "Device call aborted", "Generic error", "Cancelled by user", "Object ID too low", "Object ID too high", "Object not in heap", "Unknown heap", "Unknown object (invalid DefProc)", "Unknown object (DefProc not in table)", "Message out of range", "Invalid (null) method", "Unknown message", "Manager call not supported", "Bad address", "Network operation in progress", "Network operation timed out", "Connection is busy", "Network attribute not supported", "Network error", "Address in use", "System out of memory", "Connection aborted", "Connection refused", "Not connected", "Already connected", "Connection closed", "Initialization error (interapplication manager)", "Bad occurrence", "Wait on unbound occurrence handler", "Occurrence queue overflow", "Datalog type conflict", "Unused", "Unrecognized type (interapplication manager)", "Memory corrupt", "Failed to make temporary DLL", "Old CIN version", "Drag socket not found", "Failed to load drop-object", "Failed to register OLE object", "Failed to release OLE object", "Format specifier type mismatch", "Unknown format specifier", "Too few format specifiers", "Too many format specifiers", "Scan failed", "Newer CIN version", "Error converting to variant", "Runtime menu error", "Password tampered", "Variant attribute not found", "Incompatible variant data type", "Event data is not available", "Event Store is not present", "Occurrence is not found", "Event Queue is not created", "Event info is not available", "Refnum passed is NULL", "Error retrieving Class GUID", "Error retrieving CoClass GUID", "Error retrieving TypeLib GUID.", "Bad built application magic bytes.", "Specific driver is different from the specific driver associated with the Logical Name.", "There is no session opened to the class driver.", "Max Error", "MAX - Error with config objects", "MAX - Error loading configuration", "MAX - Group not supported"]
        # "Current State"
        # "Do not delete, rename, or modify this frame.\n(this is used to capture unhandled states and typos)"
        # "Handle mistyped state name (developer tool)"
        n104 = Format Into String(format string="Software Exception: Unhandled State \"%s\"." ("message"), error in=w208, w203) -> (resulting string=w211:string, error out=w210:errorcluster)  [unwired: 1 in]
        n105 = call <vilib>:"Error Cluster From Error Code.vi"("show call chain? (False)"=TRUE, "error in (no error)"=w210, "error message (\"\")"=w211, "error code (0)"=w212) -> ("error out"=w209:errorcluster)  [unwired: 5 in]
        n106 = call <vilib>:"Add State(s) to Queue__jki_lib_state_machine.vi"("State(s) in (\"\")"=w207) -> ("States Out"=w206:string)  [unwired: 14 in]
      }
      frame "Initialize Core Data" {
        # "Do not delete, rename, or modify this frame.\n(this is used to determine panel behavior on exit)"
        # "originally closed?"
        # "exe?"
        # "If panel starts closed or is an EXE, then close it when we exit"
        n107 = property class="VI"() -> ("Front Panel.Open"=w221:bool)  [unwired: 2 in, 2 out]
        n108 = property class="App"() -> ("App.Kind"=w220:T5)  [unwired: 2 in, 2 out]
        n109 = control-ref of="Current VI Reference"() -> (w214:refnum<vi>)
        n110 = Not(x=w221) -> (.not. x?=w218:bool)
        n111 = Equal?(x=w220, y=T5."Run Time System" ("Application:Kind")) -> (x = y?=w217:bool)
        n112 = Or(x=w218, y=w217) -> (x .or. y?=w215:bool)
        n113 = Bundle By Name(cluster=w216, "Core.Current VI Reference"=w214, "Core.Close Panel on Exit?"=w215) -> (w223:T7)
        n114 = call <vilib>:"Add State(s) to Queue__jki_lib_state_machine.vi"("State(s) in (\"\")"=w225) -> ("States Out"=w224:string)  [unwired: 14 in]
      }
      frame "Error Handler" {
        # "Unhandled Error -- Display it"
        # "Handle any errors here.\nYou can also output any states to clean-up after errors occur"
        # "Clear error"
        n115 = call <vilib>:"General Error Handler.vi"("error in (no error)"=w227) -> ()  [unwired: 10 in, 5 out]
        n116 = call <vilib>:"Add State(s) to Queue__jki_lib_state_machine.vi"("State(s) in Front (\"\")"="/* Post Error States", "State(s) in (\"\")"=w231) -> ("States Out"=w230:string)  [unwired: 13 in]
      }
      frame "Exit" {
        # "Do not put any code in this frame.\n(No errors that occur here will be handled.)"
        n117 = call <vilib>:"Add State(s) to Queue__jki_lib_state_machine.vi"("State(s) in (\"\")"=w236) -> ("States Out"=w235:string)  [unwired: 14 in]
      }
      frame "---------- Data ----------" {
        # "Do not put any code in this frame.\n(It is a separator no-op. You can make a copy of this frame to create a new Data frame)"
        n118 = call <vilib>:"Add State(s) to Queue__jki_lib_state_machine.vi"("State(s) in (\"\")"=w240) -> ("States Out"=w239:string)  [unwired: 14 in]
      }
      frame "Data: Initialize" {
        w241 = FALSE  # gaia shutter B
        w242 = FALSE  # gaia shutter A
        w243 = FALSE  # MRC trigger
        w244 = TRUE  # auto purge
        w245 = FALSE  # purge
        w246 = 0  # jet status tck
        w247 = FALSE  # Phosphor enable
        w248 = FALSE  # Wedge enable
        w249 = FALSE  # Jet enable
        w250 = FALSE  # Fire Continues Allowed
        w252 = u32 0  # Jet probe stage tck
        w251 = u32 0  # Tik2
        w253 = FALSE  # Jet trigger
        w254 = 0.0  # ACavePressure
        w255 = 0.0  # BCavePressure
        w256 = T8 {"Current VI Reference"=refnum, "Close Panel on Exit?"=FALSE}  # Core
        # "do not delete - used by framework"
        # "Expand Bundle to add new data elements to shift register data."
        # "Add new data here."
        # "Data names and types of shift register data are defined by this bundle."
        # "Initialize the shift-register data, here.\n(data names are defined by what you wire into the bundle function)"
        n119 = Bundle("Core"=w256, "BCavePressure"=w255, "ACavePressure"=w254, "Jet trigger"=w253, "Jet probe stage tck"=w252, "Tik2"=w251, "Fire Continues Allowed"=w250, "Jet enable"=w249, "Wedge enable"=w248, "Phosphor enable"=w247, "jet status tck"=w246, "purge"=w245, "auto purge"=w244, "MRC trigger"=w243, "gaia shutter A"=w242, "gaia shutter B"=w241) -> (w258:T7)  [unwired: 1 in]
        n120 = call <vilib>:"Add State(s) to Queue__jki_lib_state_machine.vi"("State(s) in (\"\")"=w260) -> ("States Out"=w259:string)  [unwired: 14 in]
      }
      frame "Data: Cleanup" {
        # "Cleanup any data and references, here.\n(this is called automatically, by the Macro: Exit)"
        n121 = Unbundle By Name(w261) -> ("Core.Current VI Reference"=w264:refnum<vi>)
        n122 = Close Reference(reference=w264, error in (no error)=w263) -> (error out=w262:errorcluster)
        n123 = call <vilib>:"Add State(s) to Queue__jki_lib_state_machine.vi"("State(s) in (\"\")"=w266) -> ("States Out"=w265:string)  [unwired: 14 in]
      }
      frame "---------- UI ----------" {
        # "Do not put any code in this frame.\n(It is a separator no-op. You can make a copy of this frame to create a new UI frame)"
        n124 = call <vilib>:"Add State(s) to Queue__jki_lib_state_machine.vi"("State(s) in (\"\")"=w270) -> ("States Out"=w269:string)  [unwired: 14 in]
      }
      frame "UI: Initialize" {
        # "Initialize the User Interface, here.\n(this is called automatically, by the Macro: Init)"
        n125 = call <vilib>:"Add State(s) to Queue__jki_lib_state_machine.vi"("State(s) in (\"\")"=w274) -> ("States Out"=w273:string)  [unwired: 14 in]
      }
      frame "UI: Cursor Set" {
        # "Argument"
        # "Set and Unset Cursor Busy.\n(Usage: \"UI: Cursor Set >> Busy|Idle\")"
        n126 = case shown="\"Idle\", Default" w275 {
          tunnel: w277 -> [w282 w284]
          tunnel: [w281 w283] -> w276
          frame "Idle", Default {
            n127 = call <vilib>:"Unset Busy.vi"("error in (no error)"=w282) -> ("error out"=w281:errorcluster)  [unwired: 10 in]
          }
          frame "Busy" {
            n128 = call <vilib>:"Set Busy.vi"("error in (no error)"=w284) -> ("error out"=w283:errorcluster)  [unwired: 9 in, 1 out]
          }
        }
        n129 = call <vilib>:"Add State(s) to Queue__jki_lib_state_machine.vi"("State(s) in (\"\")"=w280) -> ("States Out"=w279:string)  [unwired: 14 in]
      }
      frame "UI: Front Panel State" {
        # "Argument"
        # "Set Front Panel Open or Closed\n(Usage: \"UI: Front Panel State >> Open|Close\")"
        n130 = Unbundle By Name(w287) -> ("Core.Current VI Reference"=w286:refnum<vi>)
        n131 = case shown="\"Close\"" w285 {
          tunnel: w289 -> [w295 w308]
          tunnel: [w297 w309] -> w288
          tunnel: w286 -> [w296 w306]
          frame "Open", Default {
            n132 = property class="VI"(reference=w296, error in=w295) -> (reference out=w293:refnum<vi>, error out=w294:errorcluster, "Front Panel.Open"=w292:bool)
            n133 = case shown="False" w292 {
              tunnel: [w300 w303] -> w297
              tunnel: w294 -> [w299 w303]
              tunnel: w293 -> [w298 _]
              frame False {
                n134 = invoke class="VI" method="FP.Open"(reference=w298, error in=w299, "Activate"=TRUE, "State"=T6."Standard") -> (error out=w300:errorcluster)  [unwired: 1 in, 4 out]
              }
              frame True {
              }
            }
          }
          frame "Close" {
            n135 = property class="VI"(reference=w306, error in=w308) -> (reference out=w305:refnum<vi>, error out=w307:errorcluster, "Front Panel.Open"=w304:bool)
            n136 = case shown="True" w304 {
              tunnel: [w310 w313] -> w309
              tunnel: w307 -> [w310 w312]
              tunnel: w305 -> [_ w311]
              frame False {
              }
              frame True {
                n137 = invoke class="VI" method="FP.Close"(reference=w311, error in=w312) -> (error out=w313:errorcluster)  [unwired: 1 in, 2 out]
              }
            }
          }
        }
        n138 = call <vilib>:"Add State(s) to Queue__jki_lib_state_machine.vi"("State(s) in (\"\")"=w291) -> ("States Out"=w290:string)  [unwired: 14 in]
      }
      frame "---------- Macro ----------" {
        # "Do not put any code in this frame.\n(It is a separator no-op. You can make a copy of this frame to create a new Macro frame)"
        n139 = call <vilib>:"Add State(s) to Queue__jki_lib_state_machine.vi"("State(s) in (\"\")"=w317) -> ("States Out"=w316:string)  [unwired: 14 in]
      }
      frame "Macro: Initialize" {
        w318 = "Data: Initialize\nInitialize Core Data\nUI: Initialize\nUI: Front Panel State >> Open"  # Data: Initialize Initialize Core Data UI: Initialize UI: Front Panel State >> Open
        # "Initialization Macro\n(This is called once, when the VI starts)"
        n140 = call <vilib>:"Add State(s) to Queue__jki_lib_state_machine.vi"("State(s) in Front (\"\")"=w318, "State(s) in (\"\")"=w322) -> ("States Out"=w321:string)  [unwired: 13 in]
      }
      frame "Macro: Exit" {
        # "Exit Macro\n(This is called once, when the VI exits)"
        n141 = Unbundle By Name(w329) -> ("Core.Close Panel on Exit?"=w328:bool)
        n142 = Select(t="UI: Front Panel State >> Close", s=w328, f="") -> (s? t:f=w325:string)
        n143 = call <vilib>:"Add State(s) to Queue__jki_lib_state_machine.vi"("State(s) in (\"\")"=w325, "State(s) at Back (\"\")"="Data: Cleanup\nExit") -> ("States Out"=w323:string)  [unwired: 13 in]
        n144 = call <vilib>:"Add State(s) to Queue__jki_lib_state_machine.vi"("State(s) in Front (\"\")"=w323, "State(s) in (\"\")"=w332) -> ("States Out"=w331:string)  [unwired: 13 in]
      }
      frame "---------- New Category ----------" {
        # "Template Separator\n(You can make a copy of, or modify, this frame)"
        n145 = call <vilib>:"Add State(s) to Queue__jki_lib_state_machine.vi"("State(s) in (\"\")"=w336) -> ("States Out"=w335:string)  [unwired: 14 in]
      }
      frame "Action: Fire" {
        # "Your code here.\n(You can make a copy of, or modify, this frame)"
        n146 = property on="fire::10" class="Str"(error in=w338, "Val(Sgnl)"="fire>>force" ("Value (Signaling)")) -> (error out=w337:errorcluster)  [unwired: 1 in, 1 out]
        n147 = call <vilib>:"Add State(s) to Queue__jki_lib_state_machine.vi"("State(s) in (\"\")"=w342) -> ("States Out"=w341:string)  [unwired: 14 in]
      }
      frame "CheckJetTriggerAmp" {
        # "Your code here.\n(You can make a copy of, or modify, this frame)"
        n148 = Greater Or Equal?(x="internalshuttera::29", y=1.0) -> (x >= y?=w351:bool)
        n149 = Greater Or Equal?(x="internalshutterb::29", y=1.0) -> (x >= y?=w346:bool)
        n150 = Greater?(x="Amplitude.Ch AB::30", y=2.0) -> (0:w355:bool)
        n151 = Greater?(x="Amplitude.Ch AB::10", y=2.0) -> (0:w360:bool)
        n152 = case shown="True" w351 {
          tunnel: [w370 w371] -> w348
          tunnel: [w370 w371] -> w350
          frame False {
            w370 = FALSE
          }
          frame True {
            w371 = TRUE
          }
        }
        n153 = case shown="True" w346 {
          tunnel: [w368 w369] -> w343
          tunnel: [w368 w369] -> w345
          frame False {
            w368 = FALSE
          }
          frame True {
            w369 = TRUE
          }
        }
        n154 = case shown="True" w355 {
          tunnel: [w372 w373] -> w353
          tunnel: [w372 w373] -> w354
          frame False {
            w372 = FALSE
          }
          frame True {
            w373 = TRUE
          }
        }
        n155 = case shown="True" w360 {
          tunnel: [w374 w375] -> w359
          tunnel: [w374 w375] -> w358
          frame False {
            w374 = FALSE
          }
          frame True {
            w375 = TRUE
          }
        }
        n156 = local write "gaia shutter A"(w350) -> ()
        n157 = local write "gaia shutter B"(w345) -> ()
        n158 = local write "MRC trigger"(w354) -> ()
        n159 = local write "Jet trigger"(w358) -> ()
        n160 = Bundle By Name(cluster=w364, "Jet trigger"=w359, "MRC trigger"=w353, "gaia shutter A"=w348, "gaia shutter B"=w343) -> (w363:T7)
        n161 = call <vilib>:"Add State(s) to Queue__jki_lib_state_machine.vi"("State(s) in (\"\")"=w367) -> ("States Out"=w366:string)  [unwired: 14 in]
      }
      frame "CheckJetOpeningTime" {
        # "Your code here.\n(You can make a copy of, or modify, this frame)"
        n162 = Greater?(x="Delay.Ch B::10", y=1e-05) -> (0:w379:bool)
        n163 = case shown="True" w379 {
          tunnel: [w386 w387] -> w378
          tunnel: [w386 w387] -> w377
          frame False {
            w386 = FALSE
          }
          frame True {
            w387 = TRUE
          }
        }
        n164 = Bundle By Name(cluster=w382, "Jet enable"=w378) -> (w381:T7)
        n165 = local write "Jet enable"(w377) -> ()
        n166 = call <vilib>:"Add State(s) to Queue__jki_lib_state_machine.vi"("State(s) in (\"\")"=w385) -> ("States Out"=w384:string)  [unwired: 14 in]
      }
      frame "CheckProbeCamStage" {
        # "Your code here.\n(You can make a copy of, or modify, this frame)"
        n167 = property on="Position.Axis 3::7" class="DigNum (strict)"(error in=w396) -> (error out=w394:errorcluster, "Value"=w397:dbl)  [unwired: 1 in, 1 out]
        n168 = property on="Offset::20" class="DigNum (strict)"(error in=w394) -> (error out=w393:errorcluster, "Value"=w395:dbl)  [unwired: 1 in, 1 out]
        n169 = property on="Position::20" class="DigNum (strict)"() -> ("Value"=w390:dbl)  [unwired: 2 in, 2 out]
        n170 = Subtract(x=w395, y=w397) -> (x-y=w391:dbl)
        n171 = Subtract(x=w391, y=w390) -> (x-y=w388:dbl)
        n172 = Absolute Value(x=w388) -> (abs(x)=w392:dbl)
        n173 = Greater?(x=w392, y=0.1) -> (0:w400:bool)
        n174 = case shown="True" w400 {
          tunnel: w391 -> [_ w404]
          tunnel: w393 -> [w403 w406]
          tunnel: [w403 w405] -> w398
          frame False {
          }
          frame True {
            n175 = property on="Position::20" class="DigNum (strict)"(error in=w406, "Val(Sgnl)"=w404) -> (error out=w405:errorcluster)  [unwired: 1 in, 1 out]
          }
        }
        n176 = call <vilib>:"Add State(s) to Queue__jki_lib_state_machine.vi"("State(s) in (\"\")"=w402) -> ("States Out"=w401:string)  [unwired: 14 in]
      }
      frame "CheckPurgeValve" {
        # "Your code here.\n(You can make a copy of, or modify, this frame)"
        n177 = Equal?(x="SoftwareVars.Ch1::22", y=enum16{"off", "on"}."on") -> (x = y?=w410:bool)
        n178 = case shown="True" w410 {
          tunnel: [w420 w421] -> w407
          tunnel: [w420 w421] -> w411
          frame False {
            w420 = FALSE
          }
          frame True {
            w421 = TRUE
          }
        }
        n179 = Unbundle By Name(w415) -> ("Jet trigger"=w417:bool, "Jet enable"=w416:bool)
        n180 = local write "auto purge"(w411) -> ()
        n181 = case shown="True" w407 {
          tunnel: w417 -> [_ w438]
          tunnel: w416 -> [_ w437]
          tunnel: w415 -> [w427 w436]
          tunnel: [w426 w435] -> w414
          tunnel: w413 -> [w423 w432]
          tunnel: [w422 w431] -> w412
          frame False {
            n182 = property on="DO.Ch6::22" class="Enum (strict)"(error in=w423) -> (error out=w422:errorcluster, "Value"=w424:enum16{"off", "on"})  [unwired: 1 in, 1 out]
            n183 = case shown="\"on\"" w424 {
              tunnel: [w429 w430] -> w425
              tunnel: [w429 w430] -> w428
              frame "off", Default {
                w429 = FALSE
              }
              frame "on" {
                w430 = TRUE
              }
            }
            n184 = local write "purge"(w428) -> ()
            n185 = Bundle By Name(cluster=w427, "purge"=w425) -> (w426:T7)
          }
          frame True {
            n186 = And(x=w438, y=w437) -> (x .and. y?=w433:bool)
            n187 = case shown="False" w433 {
              tunnel: [w443 w453] -> w434
              tunnel: [w443 w453] -> w439
              tunnel: w432 -> [w441 w451]
              tunnel: [w444 w449] -> w431
              frame False {
                w443 = FALSE
                n188 = property on="DO.Ch6::22" class="Enum (strict)"(error in=w441) -> (error out=w440:errorcluster, "Value"=w442:enum16{"off", "on"})  [unwired: 1 in, 1 out]
                n189 = case shown="\"off\", Default" w442 {
                  tunnel: w440 -> [w445 w448]
                  tunnel: [w445 w447] -> w444
                  frame "off", Default {
                  }
                  frame "on" {
                    n190 = property on="DO.Ch6::22" class="Enum (strict)"(error in=w448, "Val(Sgnl)"=enum16{"off", "on"}."off" ("Value (Signaling)")) -> (error out=w447:errorcluster)  [unwired: 1 in, 1 out]
                  }
                }
              }
              frame True {
                w453 = TRUE
                n191 = property on="DO.Ch6::22" class="Enum (strict)"(error in=w451) -> (error out=w450:errorcluster, "Value"=w452:enum16{"off", "on"})  [unwired: 1 in, 1 out]
                n192 = case shown="\"off\", Default" w452 {
                  tunnel: w450 -> [w455 w457]
                  tunnel: [w454 w457] -> w449
                  frame "off", Default {
                    n193 = property on="DO.Ch6::22" class="Enum (strict)"(error in=w455, "Val(Sgnl)"=enum16{"off", "on"}."on" ("Value (Signaling)")) -> (error out=w454:errorcluster)  [unwired: 1 in, 1 out]
                  }
                  frame "on" {
                  }
                }
              }
            }
            n194 = Bundle By Name(cluster=w436, "purge"=w434) -> (w435:T7)
            n195 = local write "purge"(w439) -> ()
          }
        }
        n196 = call <vilib>:"Add State(s) to Queue__jki_lib_state_machine.vi"("State(s) in (\"\")"=w419) -> ("States Out"=w418:string)  [unwired: 14 in]
      }
      frame "UpdatePressure" {
        w466 = 1
        # "Your code here.\n(You can make a copy of, or modify, this frame)"
        n197 = for {
          N: w466 -> [_]
          tunnel: [w473] -> w469 mode=indexing
          tunnel: [w472] -> w458 mode=indexing
          n198 = local read "AI_mean.Channel 0::27"() -> (w473:dbl)
          n199 = Wait (ms)(milliseconds to wait=u32 2) -> ()  [unwired: 1 out]
          n200 = local read "AI_mean.Channel 1::27"() -> (w472:dbl)
        }
        n201 = Add Array Elements(numeric array=w469) -> (sum=w468:dbl)
        n202 = Divide(x=w468, y=w466) -> (x/y=w465:dbl)
        n203 = Add Array Elements(numeric array=w458) -> (sum=w467:dbl)
        n204 = call "pressure calibration.vi"("input variable"=w465) -> ("output variable"=w464:dbl)  [unwired: 10 in]
        n205 = Divide(x=w467, y=w466) -> (x/y=w463:dbl)
        n206 = call "pressure calibration.vi"("input variable"=w463) -> ("output variable"=w462:dbl)  [unwired: 10 in]
        n207 = Bundle By Name(cluster=w460, "BCavePressure"=w464, "ACavePressure"=w462) -> (w459:T7)
        n208 = call <vilib>:"Add State(s) to Queue__jki_lib_state_machine.vi"("State(s) in (\"\")"=w471) -> ("States Out"=w470:string)  [unwired: 14 in]
      }
    }
  }
